vi "External Transition.vi"(8 "error in (no error)":errorcluster, 9 "Target State":refnum<class "State.lvclass">, 10 "Context in":refnum<data-value>, 11 "State in":refnum<class "State.lvclass">) -> (0 "error out":errorcluster, 2 "Context out":refnum<data-value>, 3 "State out":refnum<class "State.lvclass">)   [LabVIEW 2024, in "State.lvlib" / "State.lvclass"]
uses:
  State.lvclass
  Context/Context/Context.lvclass
  State.lvclass/State.ctl
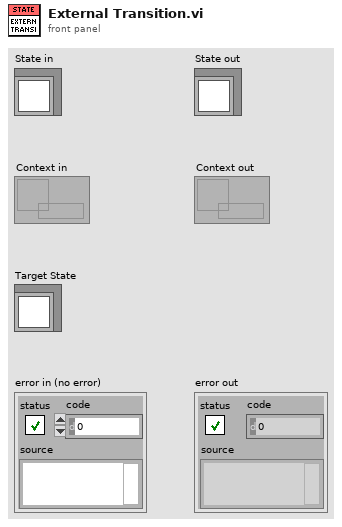
[diagram p1: front panel]
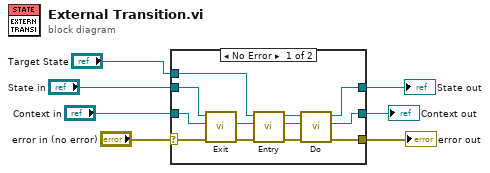
[diagram p0: block diagram]
diagram:
  n1 = case shown="No Error" "error in (no error)" {
    selector: "error in (no error)" -> [w8 w22]
    tunnel: [w11 w22] -> w6
    tunnel: [w13 w21] -> w4
    tunnel: "State in" -> [w19 w21]
    tunnel: [w12 w20] -> w3
    tunnel: "Context in" -> [w18 w20]
    tunnel: "Target State" -> [w16 _]
    frame No Error {
      n2 = call-dynamic "Exit.vi"("error in (no error)"=w8, "Context in"=w18, "State in"=w19) -> ("error out"=w9:errorcluster, "Context out"=w17:refnum<data-value>)  [unwired: 6 in, 1 out]
      n3 = call-dynamic "Entry.vi"("error in (no error)"=w9, "Context in"=w17, "State in"=w16) -> ("error out"=w10:errorcluster, "Context out"=w14:refnum<data-value>, "State out"=w15:refnum<class "State.lvclass">)  [unwired: 6 in]
      n4 = call-dynamic "Do.vi"("error in (no error)"=w10, "Context in"=w14, "State in"=w15) -> ("error out"=w11:errorcluster, "Context out"=w12:refnum<data-value>, "State out"=w13:refnum<class "State.lvclass">)  [unwired: 6 in]
    }
    frame Error {
    }
  }
  "error out" <- w6
  "State out" <- w4
  "Context out" <- w3
